vi "Periodic Tasks.vi"(8 "error in":errorcluster) -> ()   [LabVIEW 2023]
doc: "This VI runs in parallel to other tasks. It can contain as many user-defined periodic loops as you need. These can carry out PID or other sorts of timed response."
uses:
  <vilib>/Rock Robotics/WPI/DriverStation/WPI_DriverStationAllianceInfo.ctl
  <vilib>/Rock Robotics/Network Tables/NT Read String.vi
  <vilib>/Rock Robotics/Network Tables/NT Write String.vi
  GeneralPurpose/AllianceColorGlobal.vi
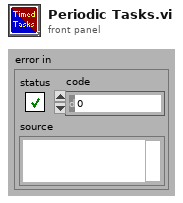
[diagram p1: front panel]
types:
  T1 = typedef "WPI_DriverStationAllianceInfo.ctl" = enum16{"Red", "Blue", "Invalid"}
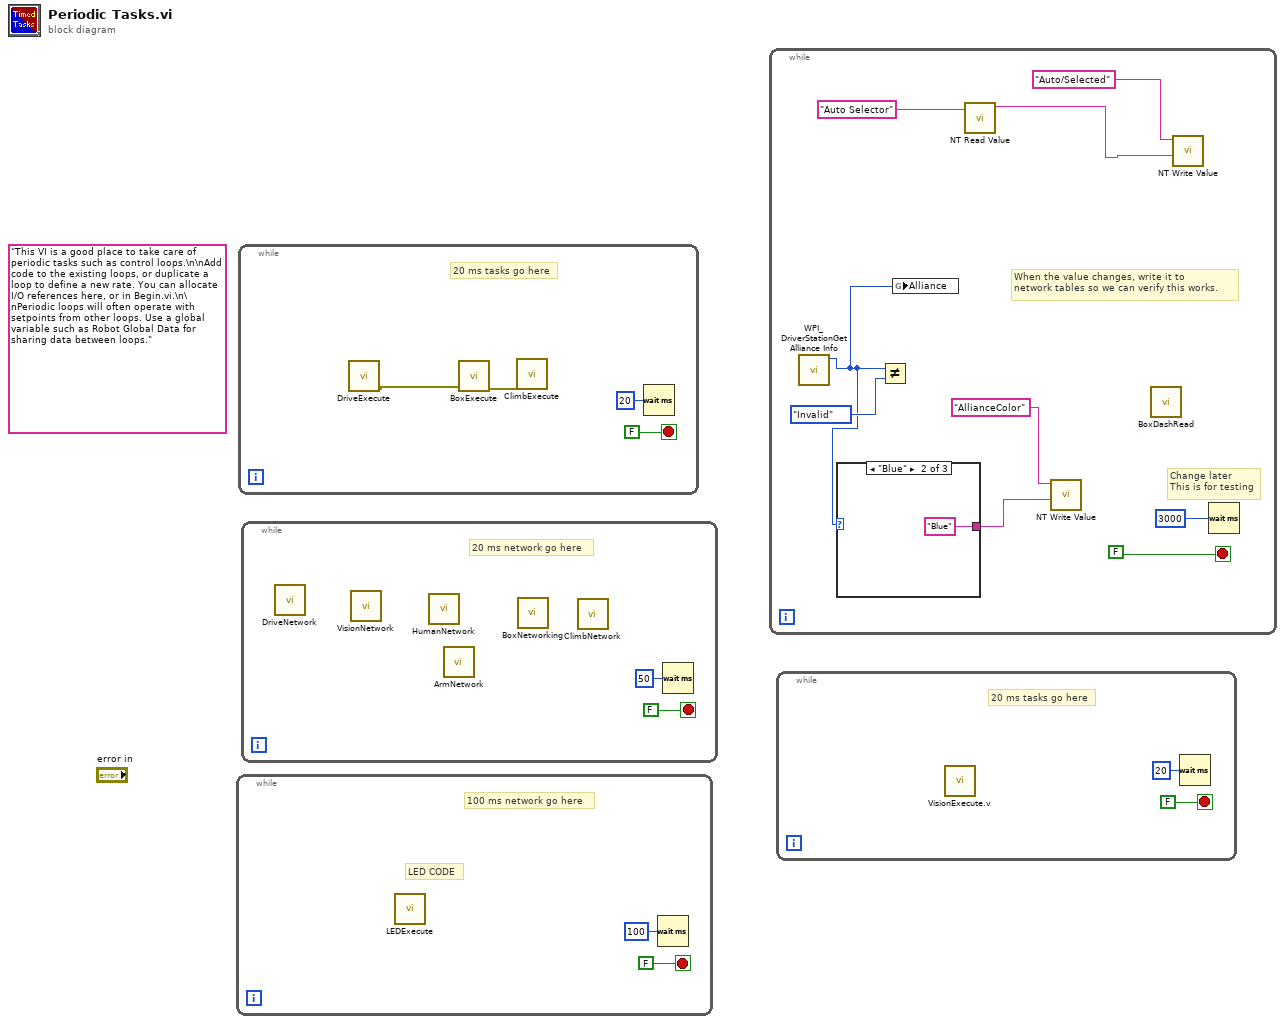
[diagram p0: block diagram]
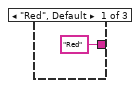
[diagram p2: hidden frame]
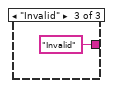
[diagram p3: hidden frame]
diagram:
  (unwired) "This VI is a good place to take care of periodic tasks such as control loops.\n\nAdd code to the existing loops, or duplicate a loop to define a new rate. You can allocate I/O references here, or in Begin.vi.\n\nPeriodic loops will often operate with setpoints from other loops. Use a global variable such as Robot Global Data for sharing data between loops."
  n1 = while {
    stop <- FALSE stop-if-true
    # "LED CODE"
    # "100 ms network go here"
    n2 = call "LEDExecute.vi"() -> ()  [unwired: 12 in]
    n3 = Wait (ms)(milliseconds to wait=u32 100) -> ()  [unwired: 1 out]
  }
  n4 = while {
    stop <- FALSE stop-if-true
    # "20 ms tasks go here"
    n5 = call "DriveExecute.vi"() -> ("error out"=w3:errorcluster)  [unwired: 11 in]
    n6 = call "BoxExecute.vi"("error in (no error)"=w3) -> ("error out"=w4:errorcluster)  [unwired: 10 in]
    n7 = call "ClimbExecute.vi"("error in (no error)"=w4) -> ()  [unwired: 10 in, 1 out]
    n8 = Wait (ms)(milliseconds to wait=u32 20) -> ()  [unwired: 1 out]
  }
  n9 = while {
    stop <- FALSE stop-if-true
    # "20 ms network go here"
    n10 = call "DriveNetwork.vi"() -> ()  [unwired: 11 in, 1 out]
    n11 = call "VisionNetwork.vi"() -> ()  [unwired: 11 in, 1 out]
    n12 = call "HumanNetwork.vi"() -> ()  [unwired: 11 in, 1 out]
    n13 = call "ArmNetwork.vi"() -> ()  [unwired: 12 in]
    n14 = call "BoxNetworking.vi"() -> ()  [unwired: 12 in]
    n15 = call "ClimbNetwork.vi"() -> ()  [unwired: 12 in]
    n16 = Wait (ms)(milliseconds to wait=u32 50) -> ()  [unwired: 1 out]
  }
  n17 = while {
    stop <- FALSE stop-if-true
    # "When the value changes, write it to \nnetwork tables so we can verify this works."
    # "Change later\nThis is for testing"
    n18 = call <vilib>:"WPI_DriverStationGet Alliance Info.vi"() -> ("Alliance"=w14:T1)  [unwired: 6 in, 5 out]
    n19 = case shown="\"Blue\"" w14 {
      tunnel: ["Red" "Blue" "Invalid"] -> w13
      frame "Red", Default {
      }
      frame "Blue" {
      }
      frame "Invalid" {
      }
    }
    n20 = Not Equal?(x=w14, y=WPI_DriverStationAllianceInfo."Invalid") -> ()  [unwired: 1 out]
    n21 = global write "AllianceColorGlobal.vi" "Alliance"(w14) -> ()
    n22 = call-poly <vilib>:"NT Read Value.vi"("name"="Auto Selector" ("Name")) -> ("value"=w9:string)  [unwired: 8 in, 2 out]
    n23 = call-poly <vilib>:"NT Write Value.vi"("value"=w13, "name"="AllianceColor") -> ()  [unwired: 9 in, 1 out]
    n24 = call "BoxDashRead.vi"() -> ()  [unwired: 12 in]
    n25 = call-poly <vilib>:"NT Write Value.vi"("value"=w9, "name"="Auto/Selected") -> ()  [unwired: 9 in, 1 out]
    n26 = Wait (ms)(milliseconds to wait=u32 3000) -> ()  [unwired: 1 out]
  }
  n27 = while {
    stop <- FALSE stop-if-true
    # "20 ms tasks go here"
    n28 = call "VisionExecute.v.vi"() -> ()  [unwired: 12 in]
    n29 = Wait (ms)(milliseconds to wait=u32 20) -> ()  [unwired: 1 out]
  }
